vi "Active Channel_AE.vi"(7 "Action":enum16{"READ", "WRITE"}(ring), 11 "Active Channel In":refnum<vi>) -> (3 "Active Channel Out":refnum<vi>)   [LabVIEW 2014]
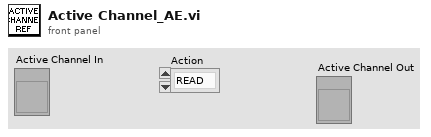
[diagram p1: front panel]
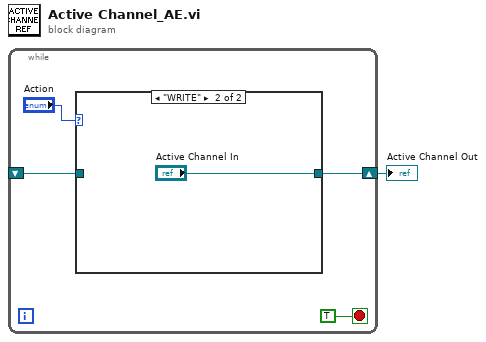
[diagram p0: block diagram]
diagram:
  n1 = while {
    shift-right: [w4] -> w1
    shift-left: _ -> [w2]
    stop <- TRUE stop-if-true
    n2 = case shown="\"WRITE\"" "Action" {
      tunnel: [w6 "Active Channel In"] -> w4
      tunnel: w2 -> [w6 _]
      frame "READ", Default {
      }
      frame "WRITE" {
      }
    }
  }
  "Active Channel Out" <- w1
